vi "LimitFunktion.vi"(7 "String":string, 9 "Boolean":bool, 11 "error in":errorcluster) -> (8 "Answer":string, 15 "error out":errorcluster)   [LabVIEW 2014, in "FH 55.lvlib"]
doc: "Die Limitfunktion vergleicht aktuelle Messwerte mit der Unter- und Obergrenze und gibt den Status als Antwort zurück (LOW, HIGH, OK).\n\n\nThe limit function compares current readings with the lower and upper limits and returns the status response (LOW, HIGH, OK)."
uses:
  FH 55.lvlib
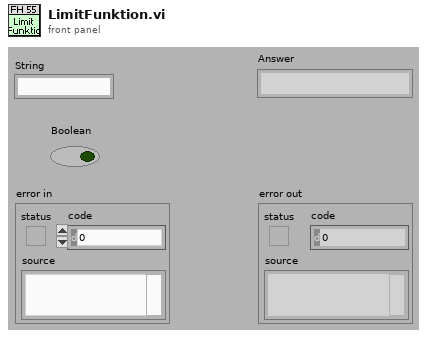
[diagram p1: front panel]
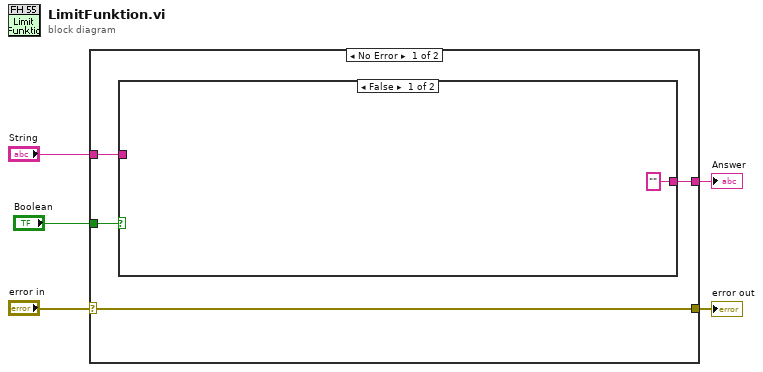
[diagram p0: block diagram]
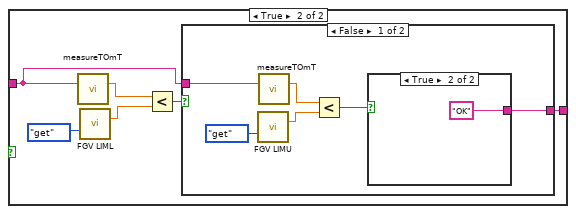
[diagram p2: hidden frame]
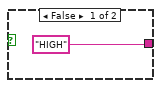
[diagram p3: hidden frame]
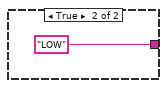
[diagram p4: hidden frame]
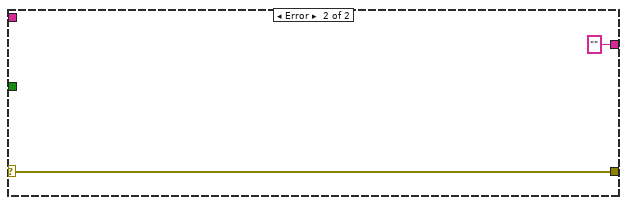
[diagram p5: hidden frame]
diagram:
  n1 = case shown="No Error" "error in" {
    selector: "error in" -> [w7 w26]
    tunnel: [w9 ""] -> w5
    tunnel: "String" -> [w8 _]
    tunnel: [w7 w26] -> w2
    tunnel: "Boolean" -> [w6 _]
    frame No Error {
      n2 = case shown="False" w6 {
        tunnel: ["" w16] -> w9
        tunnel: w8 -> [_ w11]
        frame False {
        }
        frame True {
          n3 = call "measureTOmT.vi"("string"=w11) -> ("Numeric"=w13:dbl)  [unwired: 12 in, 2 out]
          n4 = call "FGV LIML.vi"("action"=enum16{"set", "get"}."get") -> ("Numeric 2"=w12:dbl)  [unwired: 14 in]
          n5 = Less?(x=w13, y=w12) -> (x < y?=w15:bool)
          n6 = case shown="False" w15 {
            tunnel: [w21 "LOW"] -> w16
            tunnel: w11 -> [w19 _]
            frame False {
              n7 = call "FGV LIMU.vi"("action"=enum16{"set", "get"}."get") -> ("Numeric 2"=w18:dbl)  [unwired: 14 in]
              n8 = call "measureTOmT.vi"("string"=w19) -> ("Numeric"=w17:dbl)  [unwired: 12 in, 2 out]
              n9 = Less?(x=w17, y=w18) -> (x < y?=w22:bool)
              n10 = case shown="True" w22 {
                tunnel: ["HIGH" "OK"] -> w21
                frame False {
                }
                frame True {
                }
              }
            }
            frame True {
            }
          }
        }
      }
    }
    frame Error {
    }
  }
  "Answer" <- w5
  "error out" <- w2
